vi "Detailed Project Information.vi"(0 "Project  Information Input":string[][](array[string])) -> (10 "TDR Setting2":string[](array[string]), 11 "minus 2X?":bool, 14 "CMP Setting":string[](array[string]), 15 "smooth point":i32, 16 "TDR Test Item Name":string[](array[string]), 17 "Report Config":string[](array[string]), 18 "ILD Spec No":i32, 19 "Report Name":string, 20 "S-para Pair Name":string[](array[string])=["TX0", "TX1", "TX2", "TX3", "RX0", "RX1", "RX2", "RX3"], 21 "TDR Setting":string[](array[string]), 22 "NEXT Pair Name":string[](array[string])=["TX0-RX0", "TX1-RX0", "TX2-RX0", "TX3-RX0", "TX0-RX1", "TX1-RX1", "TX2-RX1", "TX3-RX1", "TX0-RX2", "TX1-RX2", "TX2-RX2", "TX3-RX2", "TX0-RX3", "TX1-RX3", "TX2-RX3", "TX3-RX3"], 23 "SingleTest Item Name":string[](array[string]), 24 "FEXT Pair Name":string[](array[string])=["TX1-RX0", "TX2-RX0", "TX3-RX0", "TX0-RX1", "TX2-RX1", "TX3-RX1", "TX0-RX2", "TX1-RX2", "TX3-RX2", "TX0-RX3", "TX1-RX3", "TX2-RX3"], 25 "Diff Test Item Name":string[](array[string])=["SDD21", "SDD22", "SCD21", "SCD22", "SCC11", "SCC22", "NEXT", "FEXT"], 26 "Spec Association Col No":string[](array[string])=["1", "2", "NAN", "NAN", "NAN", "NAN", "NAN", "NAN"], 27 "Cal File Path":string[](array[string])=["D:\\CALFILES\\cable.csa"])   [LabVIEW 2011]
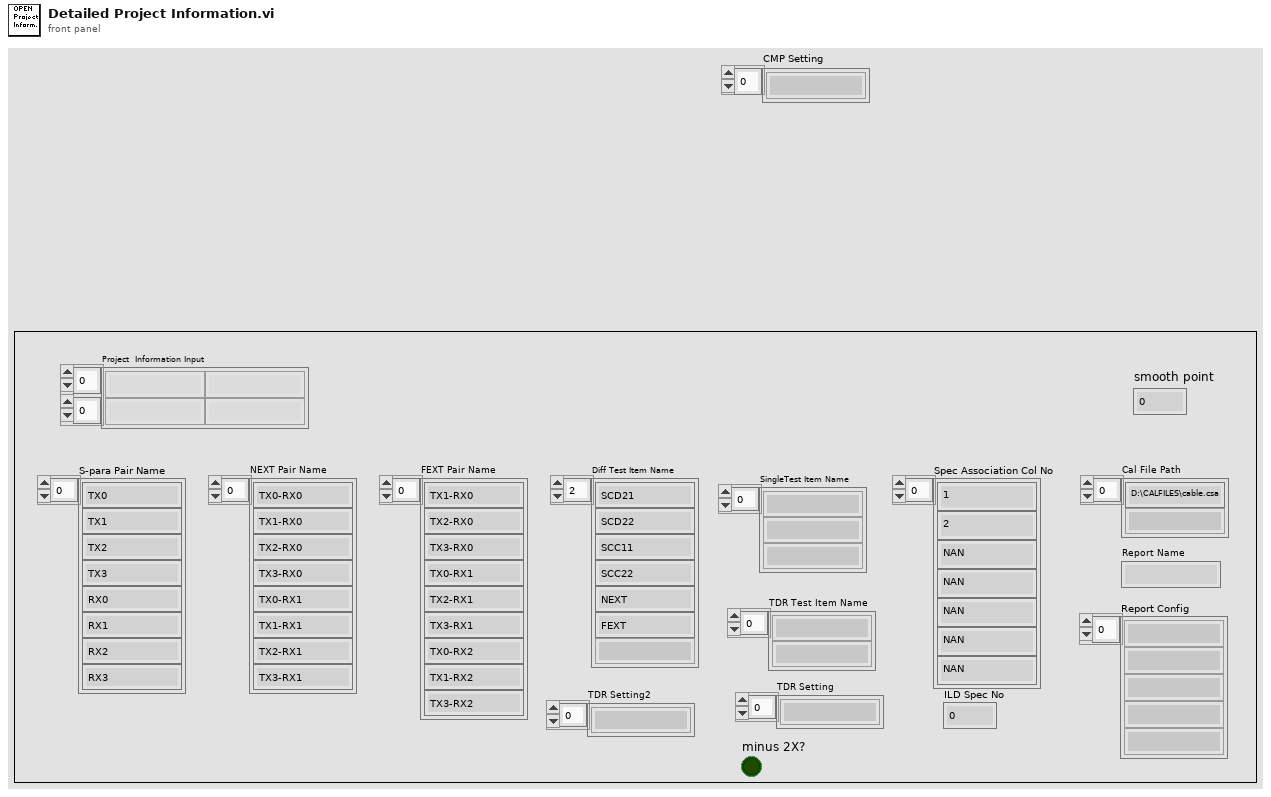
[diagram p1: front panel]
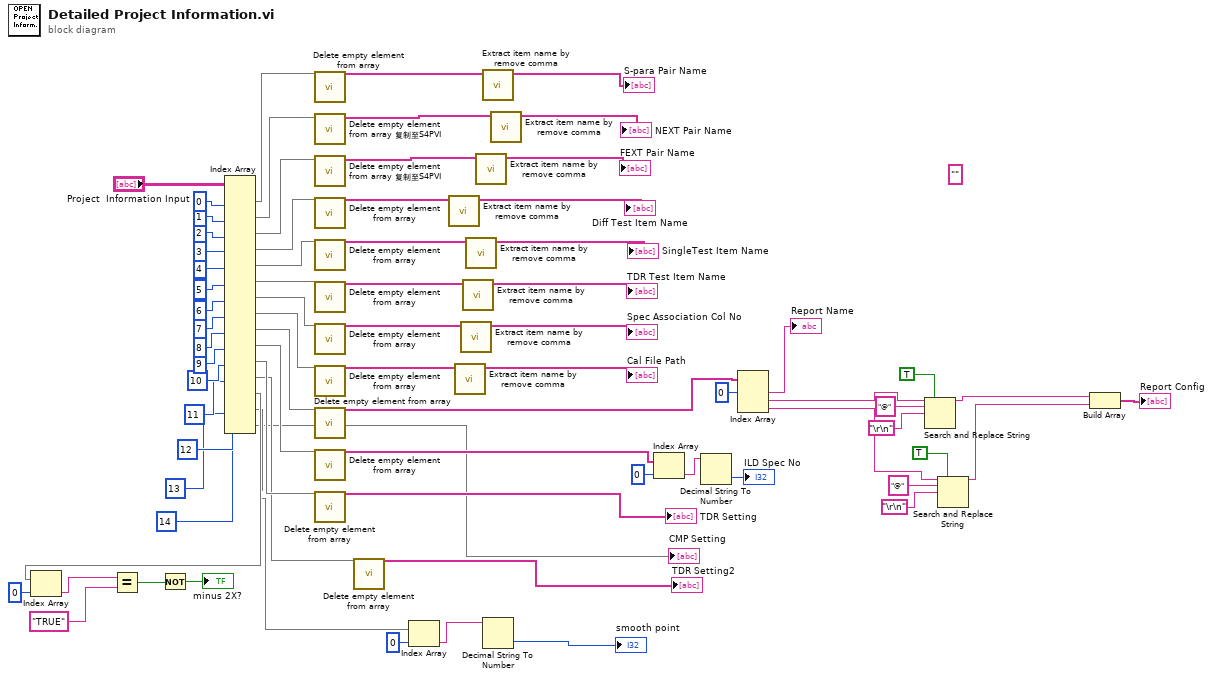
[diagram p0: block diagram]
diagram:
  (unwired) ""
  n1 = Index Array(array="Project  Information Input", index (col) #1=0 ("禁用的索引 (列)"), index (col) #2=1 ("索引 (列)"), index (col) #3=2 ("索引 (列)"), index (col) #4=3 ("索引 (列)"), index (col) #5=4 ("索引 (列)"), index (col) #6=5 ("索引 (列)"), index (col) #7=6 ("索引 (列)"), index (col) #8=7 ("索引 (列)"), index (col) #9=8 ("索引 (列)"), index (col) #10=9 ("索引 (列)"), index (col) #11=10 ("索引 (列)"), index (col) #12=11 ("索引 (列)"), index (col) #13=12 ("索引 (列)"), index (col) #14=13 ("索引 (列)"), index (col) #15=14 ("索引 (列)")) -> (element #1=w49:string[], element #2=w48:string[], element #3=w47:string[], element #4=w46:string[], element #5=w45:string[], element #6=w44:string[], element #7=w43:string[], element #8=w42:string[], element #9=w41:string[], element #10=w40:string[], element #11=w39:string[], element #12=w9:string[], element #13=w10:string[], element #14=w6:string[], element #15=→"CMP Setting":string[])  [unwired: 15 in]
  n2 = Index Array(array=w10, index=0 ("索引")) -> (element=w15:string)
  n3 = Equal?(x=w15, y="TRUE") -> (x = y?=w13:bool)
  n4 = Not(x=w13) -> (.not. x?=→"minus 2X?":bool)
  n5 = call "Delete empty element from array.vi"("Array In"=w49) -> ("Array out"=w75:string[])  [unwired: 26 in]
  n6 = call "Delete empty element from array 复制至S4PVI.vi"("input"=w48) -> ("output"=w74:string[])  [unwired: 10 in]
  n7 = call "Delete empty element from array 复制至S4PVI.vi"("input"=w47) -> ("output"=w73:string[])  [unwired: 10 in]
  n8 = call "Delete empty element from array.vi"("Array In"=w46) -> ("Array out"=w71:string[])  [unwired: 26 in]
  n9 = call "Delete empty element from array.vi"("Array In"=w45) -> ("Array out"=w69:string[])  [unwired: 26 in]
  n10 = call "Delete empty element from array.vi"("Array In"=w44) -> ("Array out"=w51:string[])  [unwired: 26 in]
  n11 = call "Delete empty element from array.vi"("Array In"=w43) -> ("Array out"=w72:string[])  [unwired: 26 in]
  n12 = call "Delete empty element from array.vi"("Array In"=w42) -> ("Array out"=w70:string[])  [unwired: 26 in]
  n13 = call "Delete empty element from array.vi"("Array In"=w41) -> ("Array out"=w37:string[])  [unwired: 26 in]
  n14 = call "Delete empty element from array.vi"("Array In"=w40) -> ("Array out"=w54:string[])  [unwired: 26 in]
  n15 = call "Delete empty element from array.vi"("Array In"=w39) -> ("Array out"=→"TDR Setting":string[])  [unwired: 26 in]
  n16 = call "Delete empty element from array.vi"("Array In"=w9) -> ("Array out"=→"TDR Setting2":string[])  [unwired: 26 in]
  n17 = Index Array(array=w6, index=0 ("索引")) -> (element=w4:string)
  n18 = call "Extract item name by remove comma .vi"("Pair  Name In"=w71) -> ("Pair Name Out"=→"Diff Test Item Name":string[])  [unwired: 10 in]
  n19 = call "Extract item name by remove comma .vi"("Pair  Name In"=w70) -> ("Pair Name Out"=→"Cal File Path":string[])  [unwired: 10 in]
  n20 = call "Extract item name by remove comma .vi"("Pair  Name In"=w72) -> ("Pair Name Out"=→"Spec Association Col No":string[])  [unwired: 10 in]
  n21 = call "Extract item name by remove comma .vi"("Pair  Name In"=w51) -> ("Pair Name Out"=→"TDR Test Item Name":string[])  [unwired: 10 in]
  n22 = call "Extract item name by remove comma .vi"("Pair  Name In"=w69) -> ("Pair Name Out"=→"SingleTest Item Name":string[])  [unwired: 10 in]
  n23 = call "Extract item name by remove comma .vi"("Pair  Name In"=w73) -> ("Pair Name Out"=→"FEXT Pair Name":string[])  [unwired: 10 in]
  n24 = call "Extract item name by remove comma .vi"("Pair  Name In"=w75) -> ("Pair Name Out"=→"S-para Pair Name":string[])  [unwired: 10 in]
  n25 = Decimal String To Number(string=w4) -> (number=→"smooth point":i32)  [unwired: 2 in, 1 out]
  n26 = call "Extract item name by remove comma .vi"("Pair  Name In"=w74) -> ("Pair Name Out"=→"NEXT Pair Name":string[])  [unwired: 10 in]
  n27 = Index Array(array=w54, index=0 ("索引")) -> (element=w53:string)
  n28 = Decimal String To Number(string=w53) -> (number=→"ILD Spec No":i32)  [unwired: 2 in, 1 out]
  n29 = Index Array(array=w37, index #1=0 ("索引")) -> (element #1=→"Report Name":string, element #2=w33:string, element #3=w28:string)  [unwired: 2 in]
  n30 = Search and Replace String(replace all?=TRUE ("替换全部？(F)"), input string=w33, search string="@", replace string="\r\n") -> (result string=w27:string)  [unwired: 4 in, 3 out]
  n31 = Search and Replace String(replace all?=TRUE ("替换全部？(F)"), input string=w28, search string="@", replace string="\r\n") -> (result string=w26:string)  [unwired: 4 in, 3 out]
  n32 = Build Array(w27, w26) -> (→"Report Config":string[])
